vi "RANGE Individual Average.vi"(6 "Avg Interval (Sec)":i32, 8 "Error In":errorcluster, 9 "Flow Rate (BTU/HR)":dbl, 11 "Array IN":dbl[](array[numeric])) -> (0 "Error Out":errorcluster, 1 "Standard Deviation (BTU/hr)":dbl format="%0.2f", 2 "Average (BTU/HR) (Out)":dbl, 3 "Array OUT":dbl[](array[numeric]))   [LabVIEW 2016]
uses:
  <vilib>/Analysis/NI_AALBase.lvlib
panel:
  out "size(s)":i32
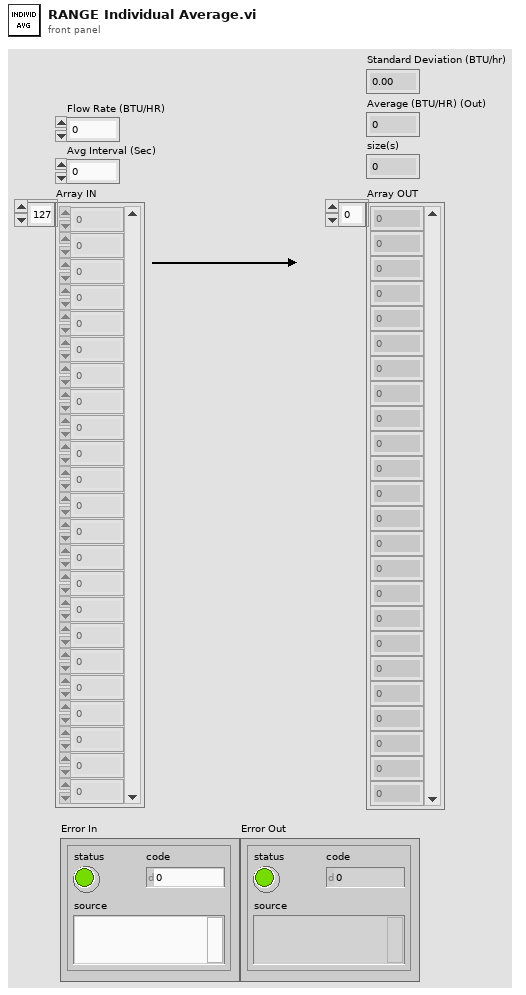
[diagram p1: front panel]
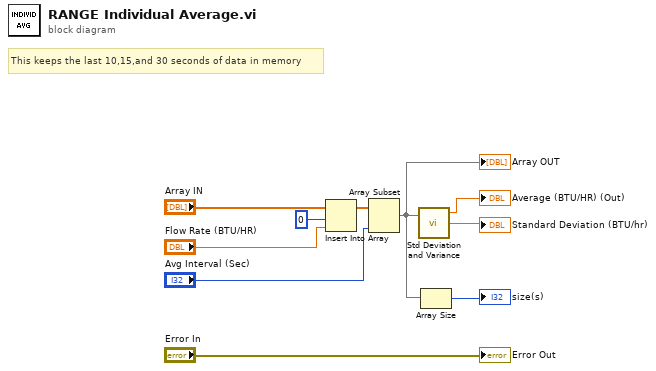
[diagram p0: block diagram]
diagram:
  # "This keeps the last 10,15,and 30 seconds of data in memory"
  n1 = Insert Into Array(array="Array IN", index=0, new element="Flow Rate (BTU/HR)") -> (w8:dbl[])
  n2 = Array Subset(array=w8, length="Avg Interval (Sec)") -> (w3:dbl[])  [unwired: 1 in]
  "Array OUT" <- w3
  n3 = call <vilib>:"Std Deviation and Variance.vi"("X"=w3) -> ("mean"=→"Average (BTU/HR) (Out)":dbl, "standard deviation"=→"Standard Deviation (BTU/hr)":dbl)  [unwired: 1 in, 1 out]
  n4 = Array Size(array=w3) -> (size(s)=→"size(s)":i32)
  "Error Out" <- "Error In"
